vi "get_number_of_channels.vi"(8 "error in (no error)":errorcluster, 11 "GenericImageAssembler.lvclass in":refnum<class "GenericImageAssembler.lvclass">) -> (0 "error out":errorcluster, 2 "number of channels":i32, 3 "GenericImageAssembler.lvclass out":refnum<class "GenericImageAssembler.lvclass">)   [LabVIEW 2010, in "GenericImageAssembler.lvclass"]
uses:
  GenericImageAssembler.lvclass
  GenericImageAssembler.lvclass/GenericImageAssembler.ctl
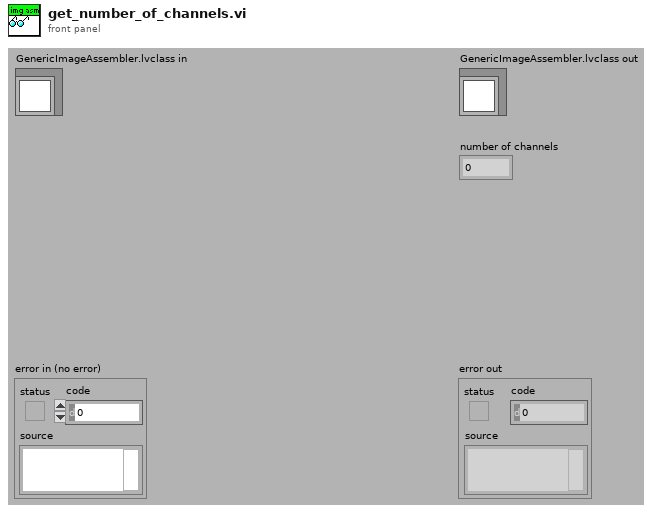
[diagram p1: front panel]
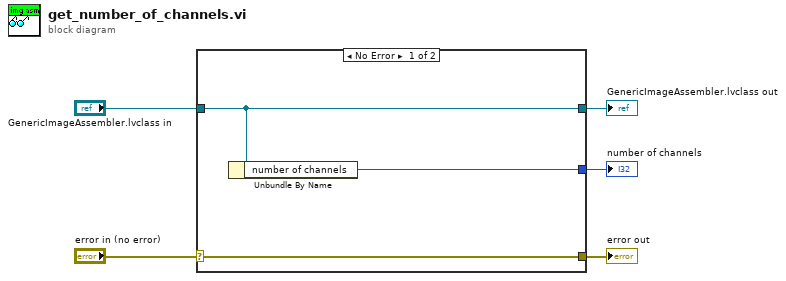
[diagram p0: block diagram]
diagram:
  n1 = case shown="No Error" "error in (no error)" {
    selector: "error in (no error)" -> [w8 w9]
    tunnel: [w8 w9] -> w4
    tunnel: [w7 w10] -> w2
    tunnel: "GenericImageAssembler.lvclass in" -> [w7 w10]
    tunnel: [w6 _] -> w1
    frame No Error {
      n2 = Unbundle By Name(w7) -> ("number of channels"=w6:i32)
    }
    frame Error {
    }
  }
  "error out" <- w4
  "GenericImageAssembler.lvclass out" <- w2
  "number of channels" <- w1
